vi "Get Session State.vi"(6 "timeout (ms)":i32=-1, 8 "error in (no error)":errorcluster, 11 "FlexLogger_gRPCAPI in":refnum<class "FlexLogger_gRPC.lvclass">) -> (0 "error out":errorcluster, 2 "Session State":T1, 3 "FlexLogger_gRPCAPI out":refnum<class "FlexLogger_gRPC.lvclass">)   [LabVIEW 2020, in "FlexLogger_gRPC.lvlib" / "FlexLogger_gRPC.lvclass"]
doc: "Gets the state of currently running flexlogger test session"
uses:
  FlexLogger_gRPC.lvclass
  Controls/FlexLogger Session State Enum.ctl
  FlexLogger_gRPC.lvclass/FlexLogger_gRPC.ctl
  FlexLogger_client/FlexLogger_client.lvlib
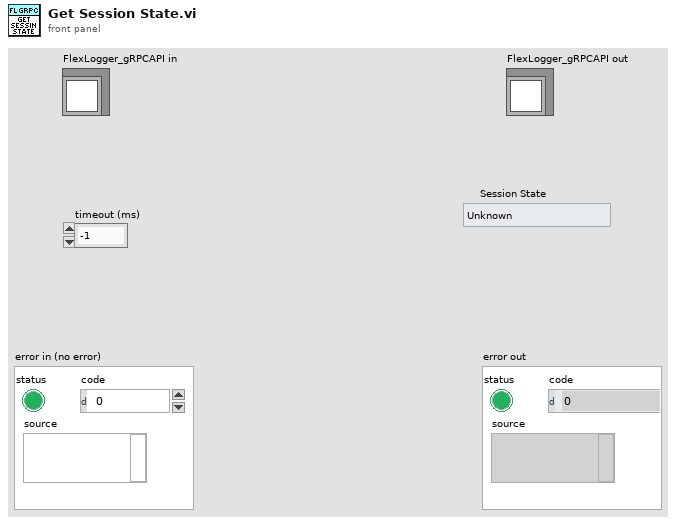
[diagram p1: front panel]
types:
  T1 = typedef "FlexLogger_gRPC.lvlib/FlexLogger_gRPC.lvclass/FlexLogger Session State Enum.ctl" = enum16{"Unknown", "Idle", "Running", "Invalid Configuration", "No Valid Logged Channels", "Paused"}
  T2 = typedef "grpc-lvsupport-release.lvlib/grpcId.ctl" = u64
  T3 = typedef "FlexLogger_client.lvlib/flexlogger_GetTestSessionStateResponse.ctl" = cluster{"test_session_state":i32}
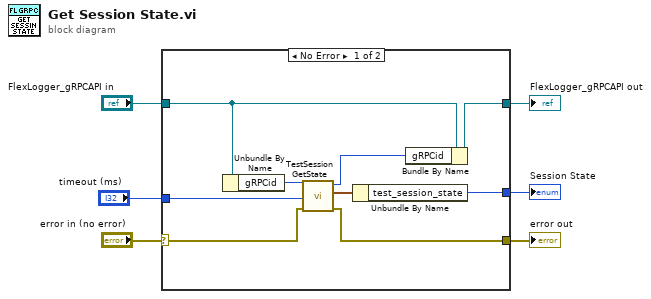
[diagram p0: block diagram]
diagram:
  n1 = case shown="No Error" "error in (no error)" {
    selector: "error in (no error)" -> [w12 w16]
    tunnel: [w14 _] -> w6
    tunnel: [w11 w16] -> w4
    tunnel: "FlexLogger_gRPCAPI in" -> [w10 w17]
    tunnel: [w9 w17] -> w2
    tunnel: "timeout (ms)" -> [w7 _]
    frame No Error {
      n2 = Unbundle By Name(w10) -> ("gRPCid"=w13:T2)
      n3 = call "TestSession GetState.vi"("error in"=w12, "timeout (ms)"=w7, "gRPC ID"=w13) -> ("error out"=w11:errorcluster, "Response Data"=w15:T3, "gRPC ID out"=w8:T2)  [unwired: 6 in]
      n4 = Unbundle By Name(w15) -> ("test_session_state"=w14:i32)
      n5 = Bundle By Name(cluster=w10, "gRPCid"=w8) -> (w9:refnum<class "FlexLogger_gRPC.lvclass">)
    }
    frame Error {
    }
  }
  "error out" <- w4
  "FlexLogger_gRPCAPI out" <- w2
  "Session State" <- w6
